vi "zadSpr_003_PH.vi"() -> ()   [LabVIEW 2021]
uses:
  <vilib>/Utility/miscctls.llb/LVTextColorsTypeDef.ctl
panel:
  out "Legend:Plot Minimum":u32
  in  "stop":bool
  out "Waveform Chart":dbl(graph)=0.0896154250709622
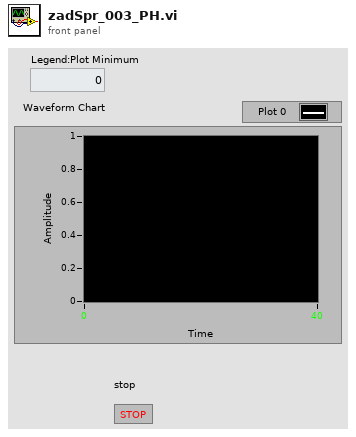
[diagram p1: front panel]
types:
  T1 = typedef "LVTextColorsTypeDef.ctl" = cluster{"Text Color":u32, "Background Color":u32}
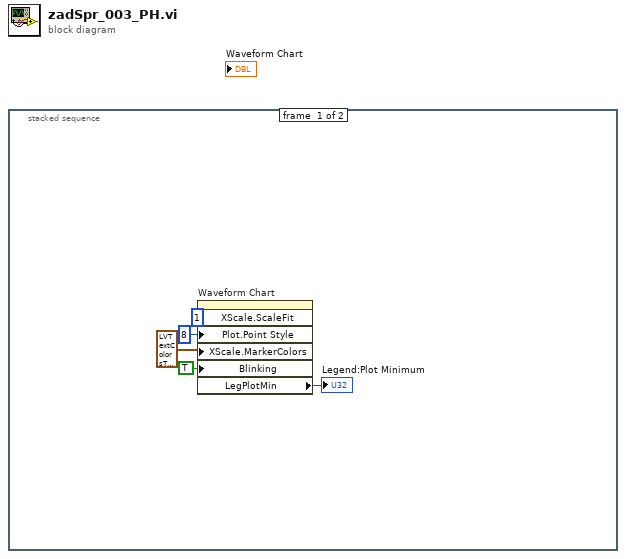
[diagram p0: block diagram]
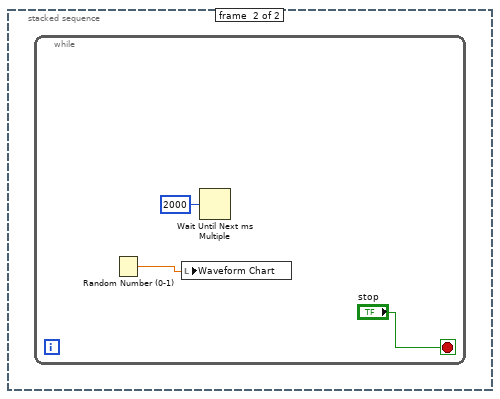
[diagram p2: hidden frame]
diagram:
  n1 = stacked-sequence {
    frame #0 {
      n2 = property on="Waveform Chart" class="WFChart (strict)"("XScale.ScaleFit"=u8 1 ("X Scale.Scale Fit"), "Plot.Point Style"=u8 8, "XScale.MarkerColors"=T1 {"Text Color"=1244928, "Background Color"=16711894} ("X Scale.Marker Colors"), "Blinking"=TRUE) -> ("LegPlotMin"=→"Legend:Plot Minimum":u32)  [unwired: 2 in, 2 out]
    }
    frame #1 {
      n3 = while {
        stop <- "stop" stop-if-true
        n4 = Random Number (0-1)() -> (number: 0 to 1=w7:dbl)
        n5 = local write "Waveform Chart"(w7) -> ()
        n6 = Wait Until Next ms Multiple(millisecond multiple=u32 2000) -> ()  [unwired: 1 out]
      }
    }
  }
